vi "test_API_1.vi"() -> ()   [LabVIEW 2014]
uses:
  message acknowledgement.ctl
  QoS levels.ctl
  MQTT client.lvclass/MQTT client.ctl
  Read connected.vi
  Read disconnect.vi
  Read QoS Ack.vi
  Read send failure.vi
  Read send success.vi
  Read subscription.vi
  Read failed to connect.vi
  MQTT client.lvclass
panel:
  out "error out":errorcluster
  in  "connect":bool
  out "subid":i32
  in  "subscribe to":string
  in  "subscribe":bool
  in  "QoS":T1=enum."At least once"
  out "send ID":i32
  out "sub_data":string
  out "sub_topic":string
  out "sub_ID":i32
  out "send failure":T2
  out "send success":T2
  out "QOS Ack":T2
  out "disconnected_message":string
  out "disconnected_code":i32
  out "connCode":i32
  out "connected":string
  in  "stop":bool
  in  "send":bool
  in  "data":string
  in  "topic":string
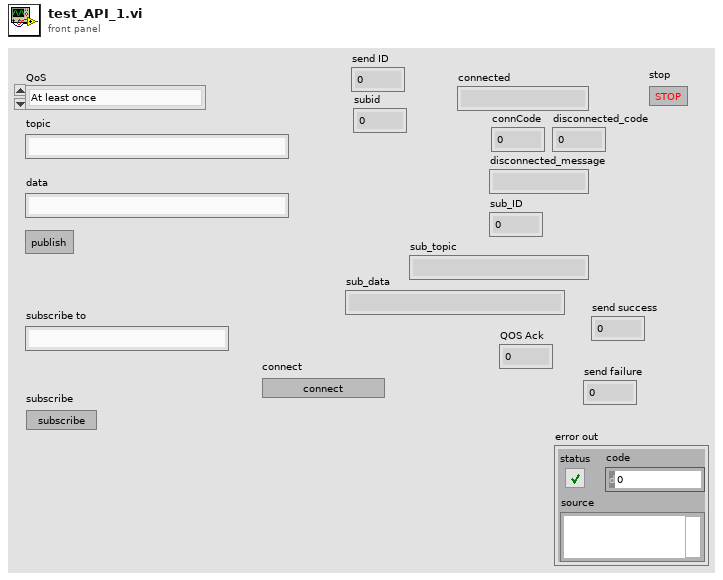
[diagram p1: front panel]
types:
  T1 = typedef "MQTT client.lvclass/QoS levels.ctl" = enum8{"None", "At least once", "Exactly once"}
  T2 = typedef "MQTT client.lvclass/message acknowledgement.ctl" = i32
  T3 = cluster{"Event Registrations:connected":refnum<event-registration>, "Event Registrations:disconnect":refnum<event-registration>, "Event Registrations:QoS Ack":refnum<event-registration>, "Event Registrations:send failure":refnum<event-registration>, "Event Registrations:send success":refnum<event-registration>, "Event Registrations:subscription":refnum<event-registration>, "Event Registrations:failed to connect":refnum<event-registration>}
  T4 = typedef "MQTT.lvlib/msgAck.ctl" = i32
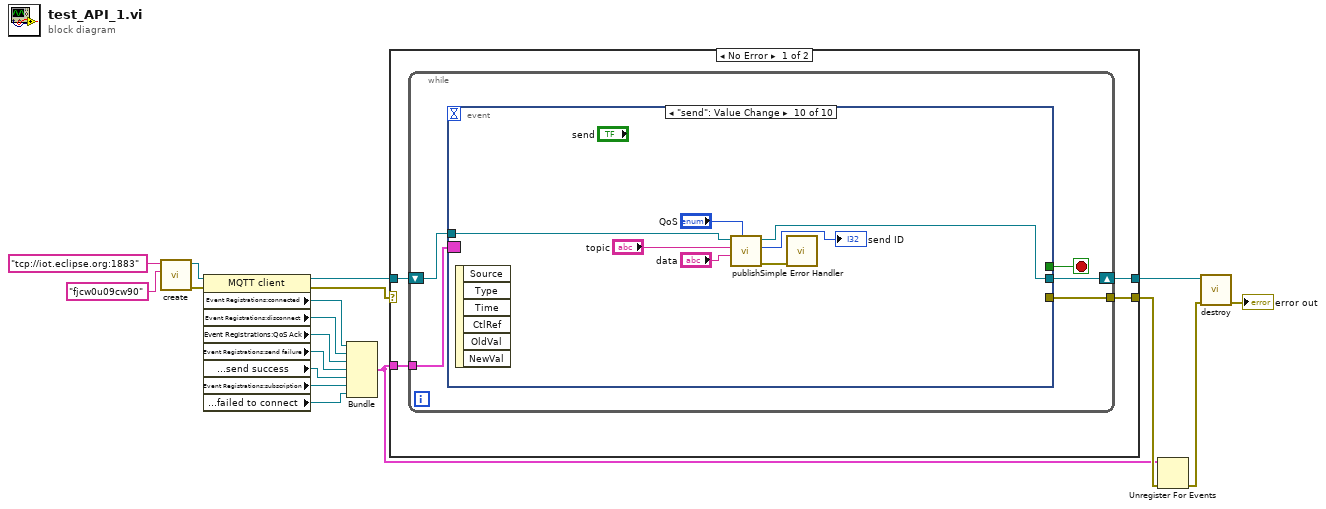
[diagram p0: block diagram]
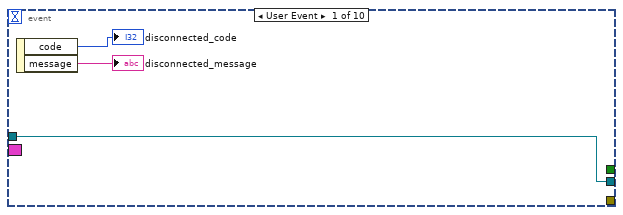
[diagram p2: hidden frame]
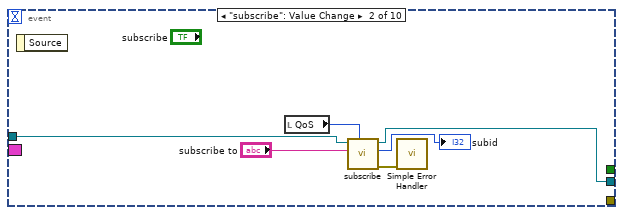
[diagram p3: hidden frame]
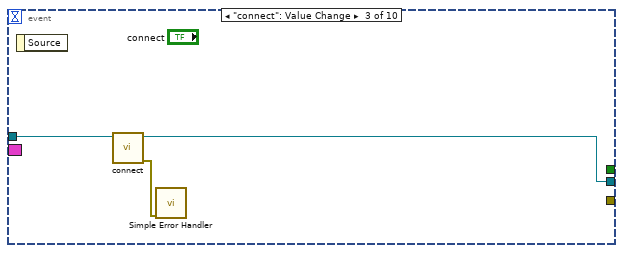
[diagram p4: hidden frame]
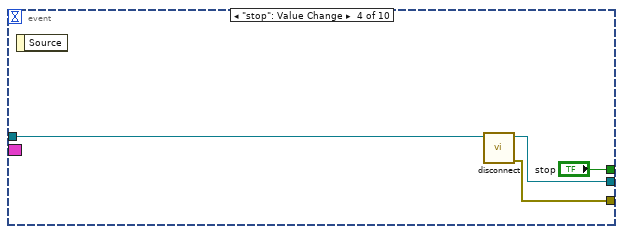
[diagram p5: hidden frame]
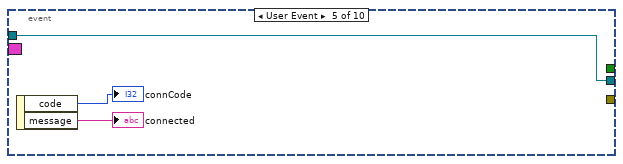
[diagram p6: hidden frame]
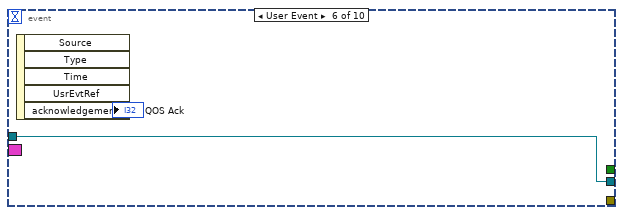
[diagram p7: hidden frame]
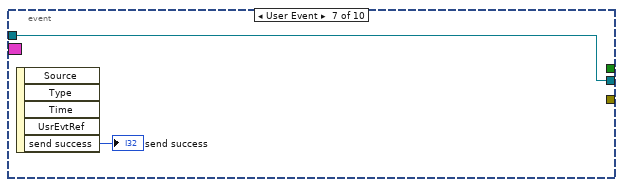
[diagram p8: hidden frame]
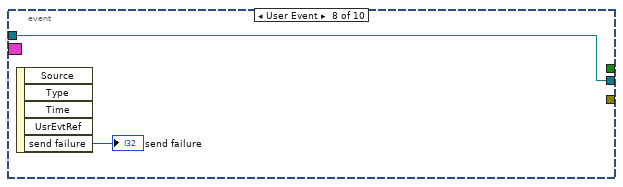
[diagram p9: hidden frame]
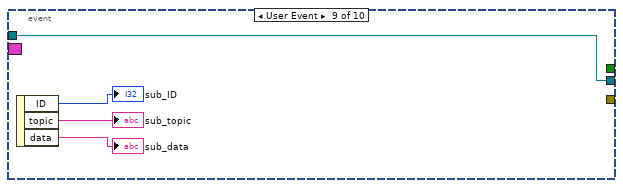
[diagram p10: hidden frame]
diagram:
  n1 = call "create.vi"("client"="fjcw0u09cw90", "URI"="tcp://iot.eclipse.org:1883") -> ("error out"=w13:errorcluster, "MQTT client out"=w11:refnum<class "MQTT client.lvclass">)  [unwired: 8 in]
  n2 = property class="MQTT client"(reference=w11, error in=w13) -> (reference out=w10:refnum<class "MQTT client.lvclass">, error out=w2:errorcluster, "Event Registrations:connected"=w9:refnum<event-registration>, "Event Registrations:disconnect"=w8:refnum<event-registration>, "Event Registrations:QoS Ack"=w7:refnum<event-registration>, "Event Registrations:send failure"=w6:refnum<event-registration>, "Event Registrations:send success"=w5:refnum<event-registration>, "Event Registrations:subscription"=w4:refnum<event-registration>, "Event Registrations:failed to connect"=w1:refnum<event-registration>)
  n3 = Bundle("Event Registrations:connected"=w9, "Event Registrations:disconnect"=w8, "Event Registrations:QoS Ack"=w7, "Event Registrations:send failure"=w6, "Event Registrations:send success"=w5, "Event Registrations:subscription"=w4, "Event Registrations:failed to connect"=w1) -> (w3:T3)  [unwired: 1 in]
  n4 = case shown="No Error" w2 {
    selector: w2 -> [_ w65]
    tunnel: w3 -> [w22 _]
    tunnel: [w19 w65] -> w18
    tunnel: w10 -> [w21 w64]
    tunnel: [w20 w64] -> w12
    frame No Error {
      n5 = while {
        tunnel: w22 -> [w27]
        shift-right: [w24] -> w20
        shift-left: w21 -> [w25]
        tunnel: [w23] -> w19
        stop <- w26 stop-if-true
        n6 = event shown="[9] \"send\": Value Change" {
          selector: w27 -> [_ _ _ _ _ _ _ _ _ _]
          dyn-events: _ -> [_ _ _ _ _ _ _ _ _ _]
          timeout: _ -> [_ _ _ _ _ _ _ _ _ _]
          tunnel: [_ _ _ "stop" _ _ _ _ _ _] -> w26
          tunnel: w25 -> [w28 w32 w38 w42 w44 w47 w49 w51 w53 w58]
          tunnel: [w28 w31 w37 w41 w44 w47 w49 w51 w53 w57] -> w24
          tunnel: [_ _ _ w40 _ _ _ _ _ _] -> w23
          event User Event {
            n7 = event-data() -> ("code"=→"disconnected_code":i32, "message"=→"disconnected_message":string)  [unwired: 1 in]
          }
          event "subscribe": Value Change {
            n8 = event-data() -> ()  [unwired: 1 in, 1 out]
            n9 = local read "QoS"() -> (w33:T1)
            n10 = call "subscribe.vi"("QoS"=w33, "topic"="subscribe to", "MQTT client in"=w32) -> ("error out"=w35:errorcluster, "request ID"=→"subid":i32, "MQTT client out"=w31:refnum<class "MQTT client.lvclass">)  [unwired: 6 in]
            n11 = call <vilib>:"Simple Error Handler.vi"("error in (no error)"=w35) -> ()  [unwired: 4 in, 5 out]
          }
          event "connect": Value Change {
            n12 = event-data() -> ()  [unwired: 1 in, 1 out]
            n13 = call "connect.vi"("MQTT client in"=w38) -> ("error out"=w39:errorcluster, "MQTT client out"=w37:refnum<class "MQTT client.lvclass">)  [unwired: 9 in]
            n14 = call <vilib>:"Simple Error Handler.vi"("error in (no error)"=w39) -> ()  [unwired: 4 in, 5 out]
          }
          event "stop": Value Change {
            n15 = event-data() -> ()  [unwired: 1 in, 1 out]
            n16 = call "disconnect.vi"("MQTT client in"=w42) -> ("error out"=w40:errorcluster, "MQTT client out"=w41:refnum<class "MQTT client.lvclass">)  [unwired: 9 in]
          }
          event User Event {
            n17 = event-data() -> ("code"=→"connCode":i32, "message"=→"connected":string)  [unwired: 1 in]
          }
          event User Event {
            n18 = event-data() -> ("acknowledgement"=→"QOS Ack":T2)  [unwired: 1 in, 4 out]
          }
          event User Event {
            n19 = event-data() -> ("send success"=→"send success":T4)  [unwired: 1 in, 4 out]
          }
          event User Event {
            n20 = event-data() -> ("send failure"=→"send failure":T4)  [unwired: 1 in, 4 out]
          }
          event User Event {
            n21 = event-data() -> ("ID"=→"sub_ID":i32, "topic"=→"sub_topic":string, "data"=→"sub_data":string)  [unwired: 1 in]
          }
          event "send": Value Change {
            n22 = event-data() -> ()  [unwired: 1 in, 6 out]
            n23 = call "publish.vi"("QoS"="QoS", "data"="data", "topic"="topic", "MQTT client in"=w58) -> ("error out"=w63:errorcluster, "send ID"=→"send ID":i32, "MQTT client out"=w57:refnum<class "MQTT client.lvclass">)  [unwired: 5 in]
            n24 = call <vilib>:"Simple Error Handler.vi"("error in (no error)"=w63) -> ()  [unwired: 4 in, 5 out]
          }
        }
      }
    }
    frame Error {
    }
  }
  n25 = Unregister For Events(event registration refnum=w3, error in=w18) -> (error out=w17:errorcluster)
  n26 = call "destroy.vi"("error in"=w17, "MQTT client in"=w12) -> ("error out"=→"error out":errorcluster)  [unwired: 9 in]
